vi "Control - Generic - Load Command Host.vi"() -> ()   [LabVIEW 2015, in "ECS-Host.lvlib"]
uses:
  ECS-Host.lvlib
  <vilib>/addons/Software Calibration Management/XControls/TBL1D.xctl
  <vilib>/addons/Software Calibration Management/XControls/SubHost.xctl
panel:
  in  "Pedal_ManE":bool
  in  "Pedal_Man":sgl caption="[]" format="%.3f"
  out "MEP_Calc":sgl caption="[bar]" format="%.3f"
  out "NominalMEP_TblOut":sgl caption="[bar]" format="%.3f"
  in  "HIG":T1(xcontrol)
  out "Pedal_Des":sgl caption="[]" format="%.3f"
  out "LoadCtrlMode":T2(ring)
  out "_IMEPGraph":cluster{"X":sgl[], "Y":sgl[]}[](graph)
  in  "LIG":T1(xcontrol)
  in  "MEP_ManE":bool
  in  "MEP_Man":sgl caption="[]" format="%.3f"
  out "MEP_Des":sgl caption="[bar]" format="%.3f"
  in  "NominalMEP_Tbl":cluster{"X":sgl[], "Y":sgl[]}(xcontrol) caption="[RPM|bar]"
  out "PedalInput":sgl caption="[%]" format="%.3f"
  out "EngineSpeed":sgl caption="[RPM]" format="%.3f"
  # "PedalOutput"
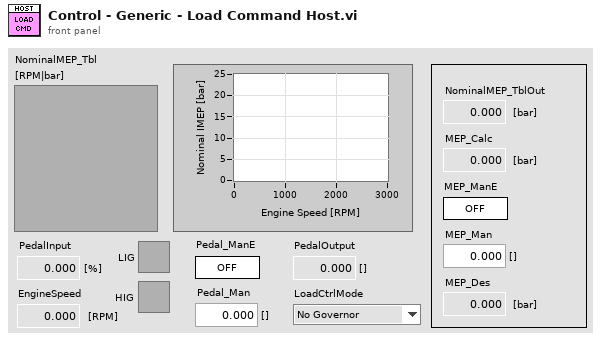
[diagram p1: front panel]
types:
  T1 = cluster{"Name":string, "Host VI":path, "Pairing File":path, "Display Name":string}
  T2 = enum32{"No Governor", "High-Idle Governor", "Low-Idle Governor"}
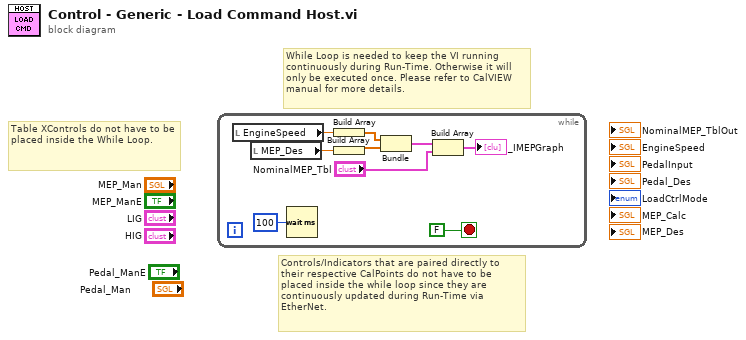
[diagram p0: block diagram]
diagram:
  # "Controls/Indicators that are paired directly to their respective CalPoints do not have to be placed inside the while loop since they are continuously updated during Run-Time via EtherNet."
  # "Table XControls do not have to be placed inside the While Loop."
  # "While Loop is needed to keep the VI running\ncontinuously during Run-Time. Otherwise it will only be executed once. Please refer to CalVIEW manual for more details."
  n1 = while {
    stop <- FALSE stop-if-true
    n2 = local read "EngineSpeed"() -> (w6:sgl)
    n3 = local read "MEP_Des"() -> (w5:sgl)
    n4 = Wait (ms)(milliseconds to wait=u32 100) -> ()  [unwired: 1 out]
    n5 = Build Array(w6) -> (w4:sgl[])
    n6 = Build Array(w5) -> (w3:sgl[])
    n7 = Bundle(w4, w3) -> (w2:cluster{sgl[], sgl[]})  [unwired: 1 in]
    n8 = Build Array(w2, "NominalMEP_Tbl") -> (→"_IMEPGraph":cluster{"X":sgl[], "Y":sgl[]}[])
  }
